vi "ESR alarms.vi"(8 "error in (no error)":errorcluster, 11 "Processing loop variables":T1 {"CurrInverter"."last updated" format="%<%H:%M\n%d/%m/%Y>T"; "CurrInverter"."set flag" items=["False", "True"]}) -> (0 "error out":errorcluster, 1 "Inv 1 over threshold?":bool[](array[boolean]), 3 "Processing loop vars out":T1 {"CurrInverter"."last updated" format="%<%H:%M\n%d/%m/%Y>T"; "CurrInverter"."set flag" items=["False", "True"]}, 4 "Inv 1 ESR":T8(array[cluster]))   [LabVIEW 2019, in "Main.lvclass"]
doc: "Developed by Kevin Thompson\nkevin@thompsonengineering.net\n\nCopyright 2020\nThompson Engineering, LLC"
uses:
  Main.lvclass
  DataTypes/Processing loop variables--cluster.ctl
  DataTypes/averaging variables.ctl
  DataTypes/ESR alarm variables.ctl
  Common/DataTypes/Inverter database record v2--cluster.ctl
  Common/DataTypes/inverter info v2--cluster.ctl
  Common/DataTypes/inverter gain range--cluster.ctl
  Common/DataTypes/inverter offset range--cluster.ctl
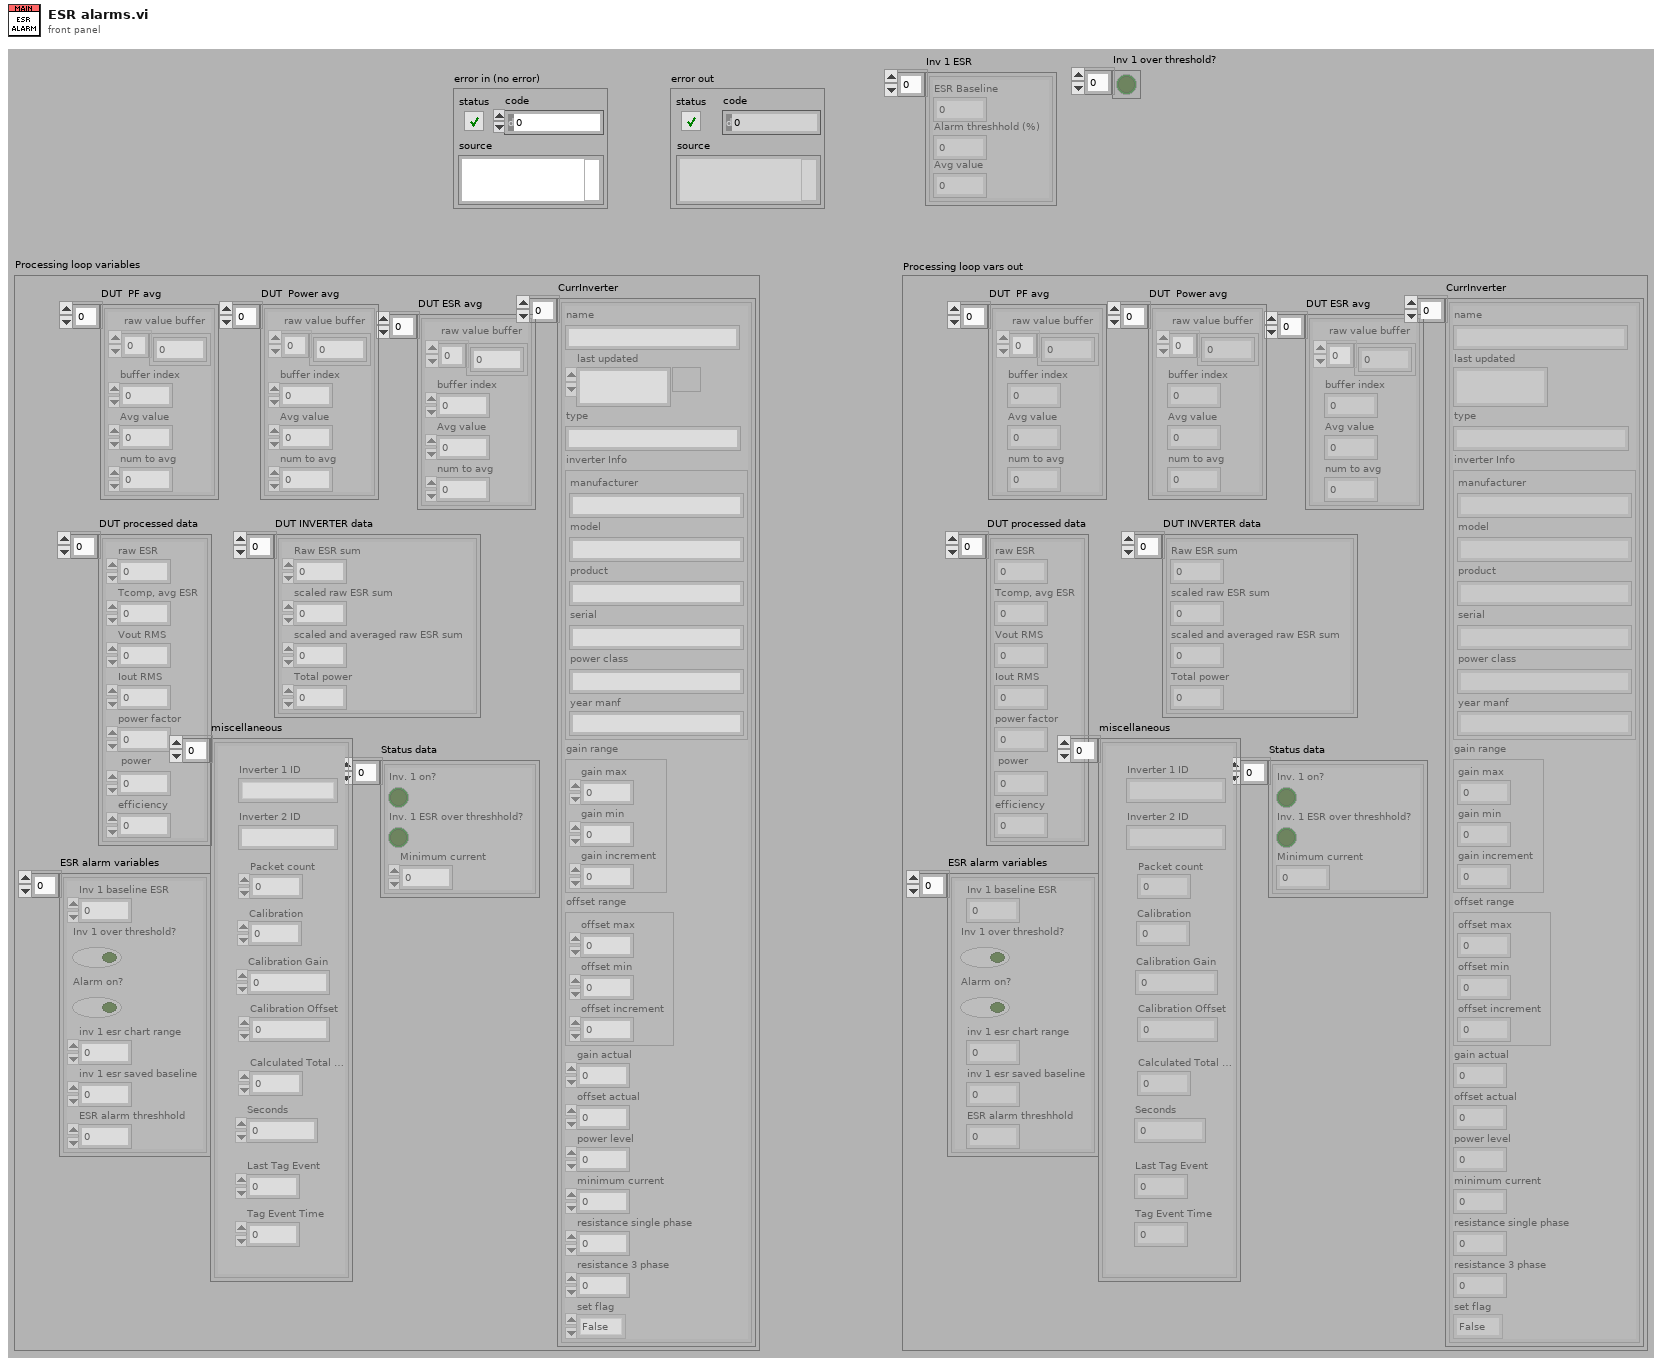
[diagram p1: front panel]
types:
  T1 = typedef "Main.lvclass/Processing loop variables--cluster.ctl" = cluster{"DUT ESR avg":T2[], "DUT  PF avg":T2[], "DUT  Power avg ":T2[], "DUT processed data":cluster{"raw ESR":dbl, "Tcomp, avg ESR":dbl, "Vout RMS":dbl, "Iout RMS":dbl, "power factor":dbl, "power":dbl, "efficiency":dbl}[], "ESR alarm variables":T3[], "Status data":cluster{"Inv. 1 on?":bool, "Inv. 1 ESR over threshhold?":bool, "Minimum current":dbl}[], "CurrInverter":T4[], "miscellaneous":cluster{"Inverter 1 ID":string, "Inverter 2 ID":string, "Packet count":u32, "Calibration":dbl, "Calibration Gain":dbl, "Calibration Offset":dbl, "Calculated Total Power":dbl, "Seconds":dbl, "Last Tag Event":dbl, "Tag Event Time":dbl}[], "DUT INVERTER data":cluster{"Raw ESR sum":dbl, "scaled raw ESR sum":dbl, "scaled and averaged raw ESR sum":dbl, "Total power":dbl}[]}
  T2 = typedef "Main.lvclass/averaging variables.ctl" = cluster{"raw value buffer":dbl[], "buffer index":i32, "Avg value":dbl, "num to avg":i32}
  T3 = typedef "Main.lvclass/ESR alarm variables.ctl" = cluster{"Inv 1 baseline ESR":dbl, "Inv 1 over threshold?":bool, "Alarm on?":bool, "inv 1 esr chart range":dbl, "inv 1 esr saved baseline":dbl, "ESR alarm threshhold":dbl}
  T4 = typedef "Inverter database record v2--cluster.ctl" = cluster{"name":string, "last updated":timestamp, "type":string, "inverter Info":T5, "gain range":T6, "offset range":T7, "gain actual":dbl, "offset actual":dbl, "power level":dbl, "minimum current":dbl, "resistance single phase":dbl, "resistance 3 phase":dbl, "set flag":u16}
  T5 = typedef "inverter info v2--cluster.ctl" = cluster{"manufacturer":string, "model":string, "product":string, "serial":string, "power class":string, "year manf":string}
  T6 = typedef "inverter gain range--cluster.ctl" = cluster{"gain max":dbl, "gain min":dbl, "gain increment":dbl}
  T7 = typedef "inverter offset range--cluster.ctl" = cluster{"offset max":dbl, "offset min":dbl, "offset increment":dbl}
  T8 = cluster{"ESR Baseline":dbl, "Alarm threshhold (%)":dbl, "Avg value":dbl}[]
  T9 = cluster{"ESR Baseline":dbl, "Alarm threshhold (%)":dbl, "Avg value":dbl}
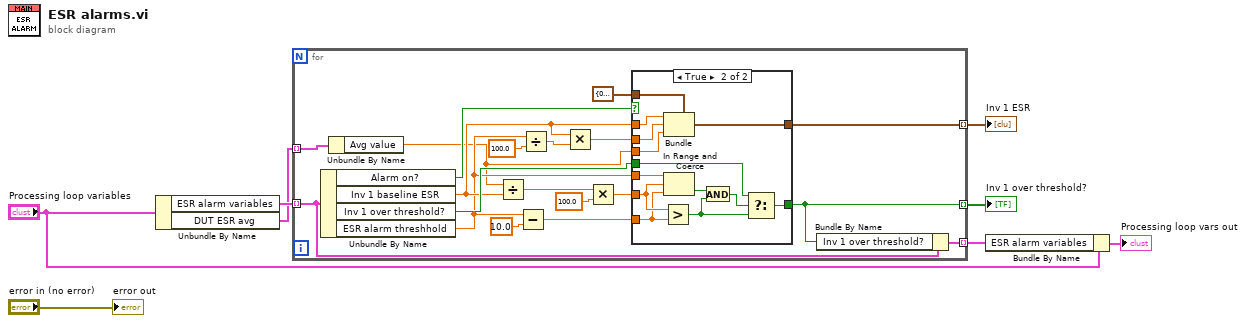
[diagram p0: block diagram]
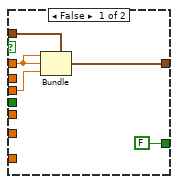
[diagram p2: hidden frame]
diagram:
  n1 = Unbundle By Name("Processing loop variables") -> ("ESR alarm variables"=w5:T3[], "DUT ESR avg"=w4:T2[])
  n2 = for {
    tunnel: [w24] -> w8 mode=indexing
    tunnel: [w22] -> w7 mode=indexing
    tunnel: w5 -> [w19] mode=indexing
    tunnel: [w18] -> w2 mode=indexing
    tunnel: w4 -> [w10] mode=indexing
    n3 = Unbundle By Name(w19) -> ("Alarm on?"=w16:bool, "Inv 1 baseline ESR"=w15:dbl, "Inv 1 over threshold?"=w20:bool, "ESR alarm threshhold"=w14:dbl)
    n4 = Unbundle By Name(w10) -> ("Avg value"=w9:dbl)
    n5 = Divide(x=w9, y=w15) -> (x/y=w27:dbl)
    n6 = Subtract(x=w14, y=10.0) -> (x-y=w23:dbl)
    n7 = Divide(x=w14, y=100.0) -> (x/y=w12:dbl)
    n8 = Multiply(x=w15, y=w12) -> (x*y=w17:dbl)
    n9 = Multiply(x=w27, y=100.0) -> (x*y=w21:dbl)
    n10 = case shown="True" w16 {
      tunnel: w14 -> [_ w38]
      tunnel: w23 -> [_ w44]
      tunnel: w21 -> [_ w45]
      tunnel: w20 -> [_ w42]
      tunnel: [FALSE ("Inv 1 over threshold?") w41] -> w24
      tunnel: [w29 w37] -> w22
      tunnel: w9 -> [w31 w36]
      tunnel: w17 -> [_ w35]
      tunnel: w15 -> [w30 w34]
      tunnel: T9 {"ESR Baseline"=0.0, "Alarm threshhold (%)"=0.0, "Avg value"=0.0} ("Inv 1 ESR") -> [w28 w33]
      frame False {
        n11 = Bundle(cluster=w28, "ESR Baseline"=w30, "Alarm threshhold (%)"=w30, "Avg value"=w31) -> (w29:T9)
      }
      frame True {
        n12 = Greater?(x=w45, y=w44) -> (0:w39:bool)
        n13 = Bundle(cluster=w33, "ESR Baseline"=w34, "Alarm threshhold (%)"=w35, "Avg value"=w36) -> (w37:T9)
        n14 = In Range and Coerce(upper limit=w38, x=w45, lower limit=w44) -> (In Range?=w40:bool)  [unwired: 1 out]
        n15 = And(x=w40, y=w39) -> (x .and. y?=w43:bool)
        n16 = Select(t=w42, s=w43, f=w39) -> (s? t:f=w41:bool)
      }
    }
    n17 = Bundle By Name(cluster=w19, "Inv 1 over threshold?"=w24) -> (w18:T3)
  }
  "Inv 1 over threshold?" <- w8
  "Inv 1 ESR" <- w7
  n18 = Bundle By Name(cluster="Processing loop variables", "ESR alarm variables"=w2) -> (→"Processing loop vars out":T1)
  "error out" <- "error in (no error)"
